vi "Launch Nested Actors.vi"(8 "error in (no error)":errorcluster, 11 "Car Wash Controller Actor in":refnum<class "Car Wash Controller Actor.lvclass">) -> (0 "error out":errorcluster, 3 "Car Wash Controller Actor out":refnum<class "Car Wash Controller Actor.lvclass">)   [LabVIEW 2019, in "Car Wash Controller Actor.lvlib" / "Car Wash Controller Actor.lvclass"]
uses:
  Car Wash Controller Actor.lvclass
  C:/Program Files (x86)/National Instruments/LabVIEW 2019/vi.lib/ActorFramework/Actor/Actor.lvclass
  Sim Entry Console Actor/Sim Entry Console Actor/Simulated Entry Console Actor.lvclass
  Simulated Wash Display Console Actor/Simulated Wash Display Console Actor/Simulated Wash Display Console Actor.lvclass
  Vehicle Position Simulation/Vehicle Position Simulation/Vehicle Position Simulation.lvclass
  Simulated Configuration Database Actor/Simulated Configuration Database Actor/Configuration Database Actor.lvclass
  Car Wash Controller Actor.lvclass/Car Wash Controller Actor.ctl
  <vilib>/ActorFramework/Actor/Actor.lvclass
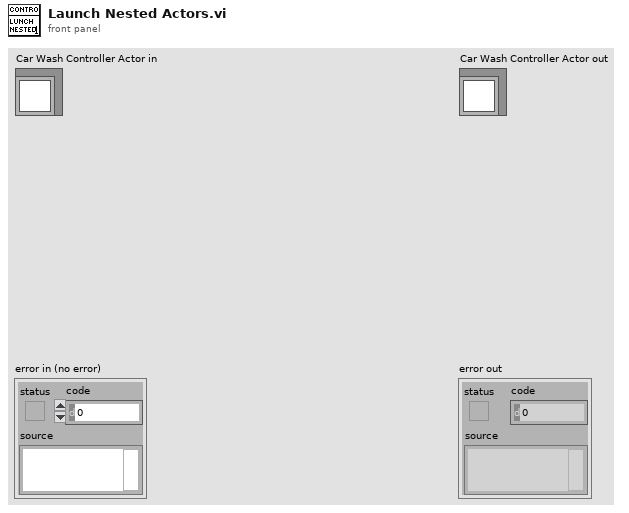
[diagram p1: front panel]
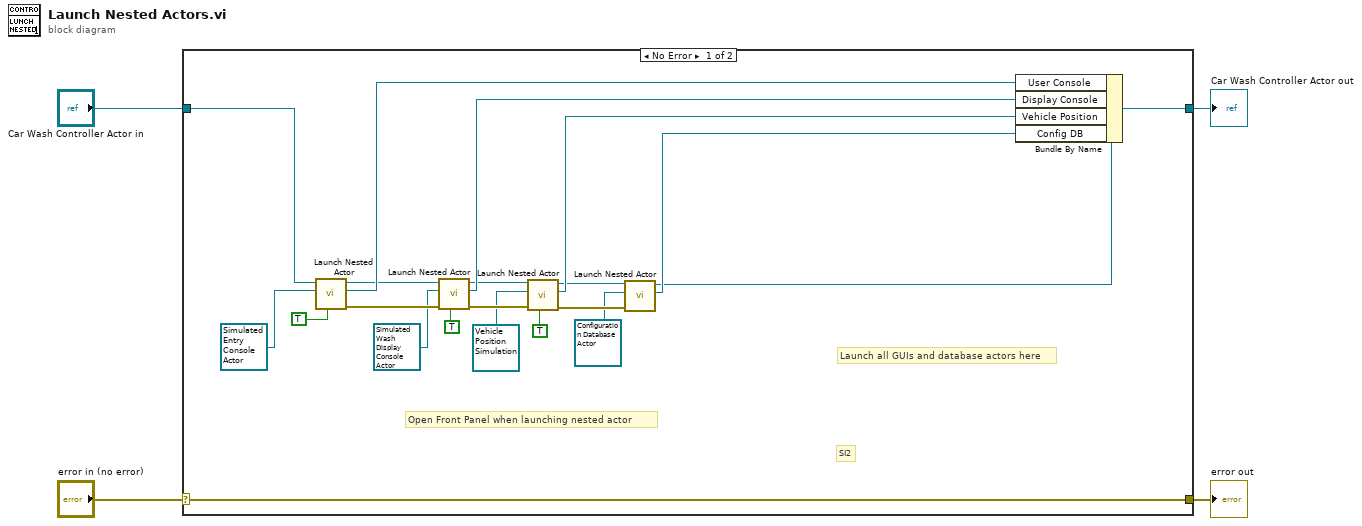
[diagram p0: block diagram]
diagram:
  n1 = case shown="No Error" "error in (no error)" {
    selector: "error in (no error)" -> [w25 w27]
    tunnel: [w25 w27] -> w3
    tunnel: [w21 w26] -> w1
    tunnel: "Car Wash Controller Actor in" -> [w22 w26]
    frame No Error {
      # "Open Front Panel when launching nested actor"
      # "Launch all GUIs and database actors here"
      # "SI2"
      n2 = call <vilib>:"Launch Nested Actor.vi"("Open Actor Core front panel? (F)"=TRUE, "Nested Actor"=refnum<class "Simulated Entry Console Actor.lvclass"> refnum ("Simulated Entry Console Actor.lvlib:Simulated Entry Console Actor.lvclass"), "Caller Actor in"=w22) -> ("error out"=w18:errorcluster, "Nested Actor's Enqueuer"=w23:refnum<class "Message Enqueuer.lvclass">, "Caller Actor out"=w19:refnum<class "Car Wash Controller Actor.lvclass">)  [unwired: 6 in]
      n3 = call <vilib>:"Launch Nested Actor.vi"("Open Actor Core front panel? (F)"=TRUE, "error in (no error)"=w18, "Nested Actor"=refnum<class "Simulated Wash Display Console Actor.lvclass"> refnum ("Simulated Wash Display Console Actor.lvlib:Simulated Wash Display Console Actor.lvclass"), "Caller Actor in"=w19) -> ("error out"=w15:errorcluster, "Nested Actor's Enqueuer"=w16:refnum<class "Message Enqueuer.lvclass">, "Caller Actor out"=w13:refnum<class "Car Wash Controller Actor.lvclass">)  [unwired: 5 in]
      n4 = call <vilib>:"Launch Nested Actor.vi"("Open Actor Core front panel? (F)"=TRUE, "error in (no error)"=w15, "Nested Actor"=refnum<class "Vehicle Position Simulation.lvclass"> refnum ("Vehicle Position Simulation.lvlib:Vehicle Position Simulation.lvclass"), "Caller Actor in"=w13) -> ("error out"=w10:errorcluster, "Nested Actor's Enqueuer"=w11:refnum<class "Message Enqueuer.lvclass">, "Caller Actor out"=w9:refnum<class "Car Wash Controller Actor.lvclass">)  [unwired: 5 in]
      n5 = call <vilib>:"Launch Nested Actor.vi"("error in (no error)"=w10, "Nested Actor"=refnum<class "Configuration Database Actor.lvclass"> refnum ("Simulated Configuration Database Actor.lvlib:Simulated Configuration Database Actor.lvclass"), "Caller Actor in"=w9) -> ("Nested Actor's Enqueuer"=w8:refnum<class "Message Enqueuer.lvclass">, "Caller Actor out"=w6:refnum<class "Car Wash Controller Actor.lvclass">)  [unwired: 6 in, 1 out]
      n6 = Bundle By Name(cluster=w6, "User Console"=w23, "Display Console"=w16, "Vehicle Position"=w11, "Config DB"=w8) -> (w21:refnum<class "Car Wash Controller Actor.lvclass">)
    }
    frame Error {
    }
  }
  "error out" <- w3
  "Car Wash Controller Actor out" <- w1
